vi "fgv_tcp_con_param.vi"(7 "tcp_connected_set":bool, 8 "Error in":errorcluster, 9 "mode":string(combo)="Get", 10 "port_set":u16, 11 "ip_address_set":string) -> (0 "error out":errorcluster, 2 "port_get":u16, 3 "ip_address_get":string, 5 "tcp_connected_get":bool)   [LabVIEW 2025]
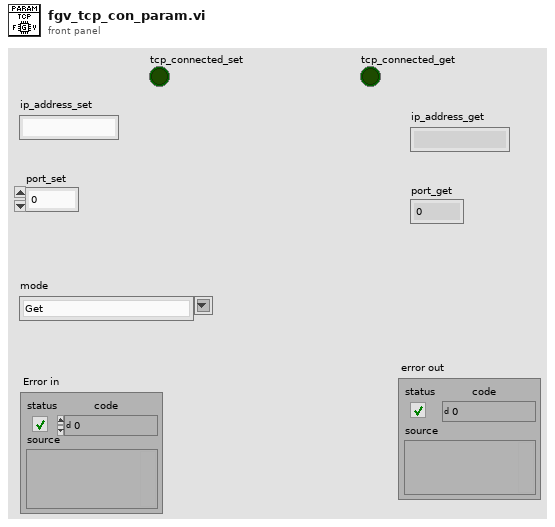
[diagram p1: front panel]
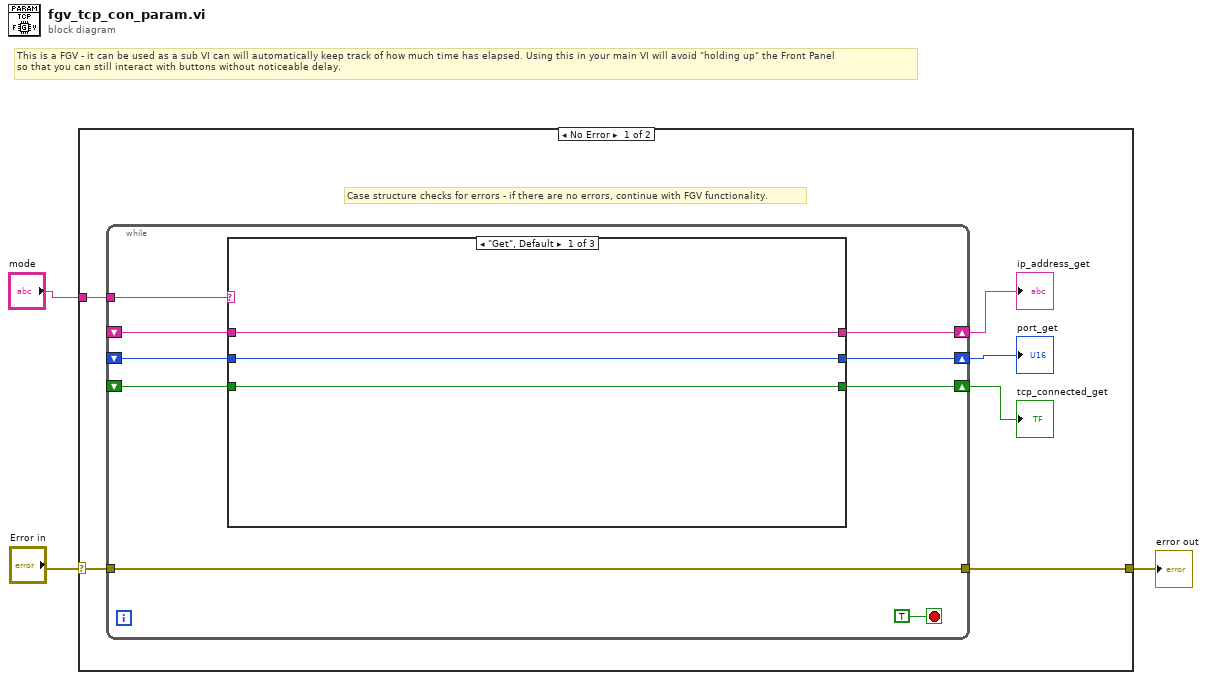
[diagram p0: block diagram]
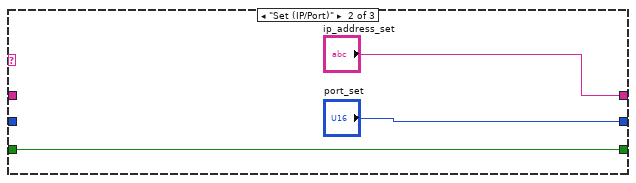
[diagram p2: hidden frame]
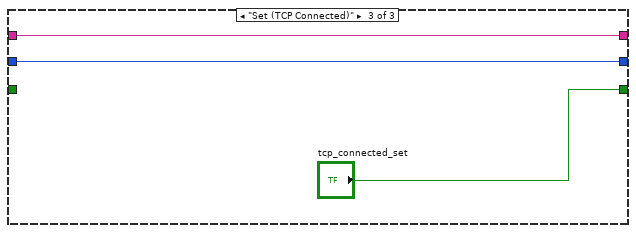
[diagram p3: hidden frame]
diagram:
  # "This is a FGV - it can be used as a sub VI can will automatically keep track of how much time has elapsed. Using this in your main VI will avoid \"holding up\" the Front Panel \nso that you can still interact with buttons without noticeable delay."
  n1 = case shown="No Error" "Error in" {
    selector: "Error in" -> [w9 w28]
    tunnel: [w8 w28] -> w2
    tunnel: "mode" -> [w7 _]
    frame No Error {
      # "Case structure checks for errors - if there are no errors, continue with FGV functionality."
      n2 = while {
        shift-right: [w17] -> w6
        shift-left: _ -> [w18]
        shift-right: [w16] -> w5
        shift-left: _ -> [w15]
        tunnel: w9 -> [w14]
        tunnel: [w14] -> w8
        tunnel: w7 -> [w13]
        shift-right: [w11] -> w4
        shift-left: _ -> [w10]
        stop <- TRUE stop-if-true
        n3 = case shown="\"Get\", Default" w13 {
          tunnel: w18 -> [w21 _ w26]
          tunnel: [w21 "ip_address_set" w26] -> w17
          tunnel: [w20 "port_set" w25] -> w16
          tunnel: w15 -> [w20 _ w25]
          tunnel: [w19 w23 "tcp_connected_set"] -> w11
          tunnel: w10 -> [w19 w23 _]
          frame "Get", Default {
          }
          frame "Set (IP/Port)" {
          }
          frame "Set (TCP Connected)" {
          }
        }
      }
      "ip_address_get" <- w6
      "port_get" <- w5
      "tcp_connected_get" <- w4
    }
    frame Error {
      # "Case structure checks for errors - if there's an errorr, do nothing except pass the error back out"
    }
  }
  "error out" <- w2
